vi "AH2500_enable_continious.vi"(3 "error in (no error)":errorcluster caption="Fehler (Eingang, kein Fehler)", 5 "AH2500-visa-address":refnum<visa-resource-name>) -> (0 "error out":errorcluster caption="Fehler (Ausgang)", 2 "AH2500-visa-address-dup":refnum<visa-resource-name>)   [LabVIEW 2018]
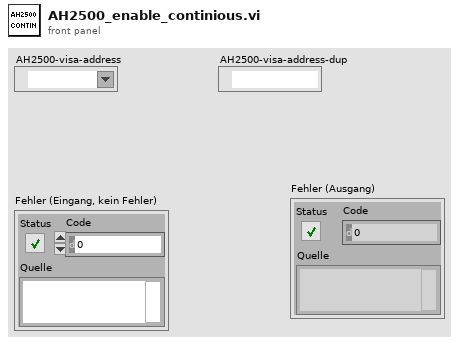
[diagram p1: front panel]
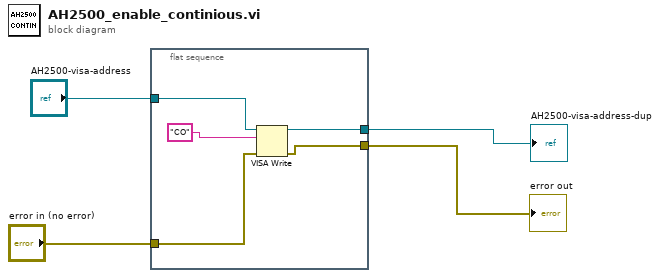
[diagram p0: block diagram]
diagram:
  n1 = flat-sequence {
    tunnel: "AH2500-visa-address" -> [w9]
    tunnel: "error in (no error)" -> [w8]
    tunnel: [w6] -> w2
    tunnel: [w5] -> w1
    frame #0 {
      n2 = VISA Write(VISA resource name=w9, write buffer="CO", error in (no error)=w8) -> (VISA resource name out=w5:refnum<visa-resource-name>, error out=w6:errorcluster)  [unwired: 1 out]
    }
  }
  "error out" <- w2
  "AH2500-visa-address-dup" <- w1
